vi "json To Minimized String - string path.vi"(8 "error in (no error)":errorcluster, 10 "path":string, 11 "JSON Document in":refnum<class "JSON Document.lvclass">) -> (0 "error out":errorcluster, 2 "json string":string, 3 "JSON Document out":refnum<class "JSON Document.lvclass">)   [LabVIEW 2015, in "JSON Document.lvclass"]
uses:
  JSON Document.lvclass
  JSON Document.lvclass/JSON Document.ctl
  rapidjson wrapper/rapidjson wrapper.lvlib
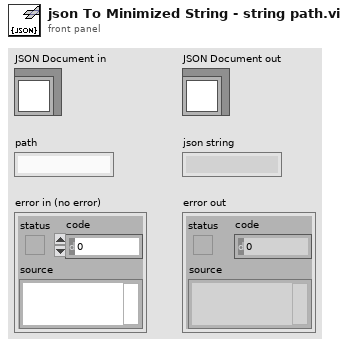
[diagram p1: front panel]
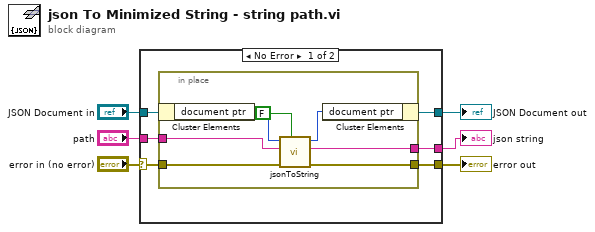
[diagram p0: block diagram]
diagram:
  n1 = case shown="No Error" "error in (no error)" {
    selector: "error in (no error)" -> [w9 w21]
    tunnel: [w8 w21] -> w5
    tunnel: [w11 w20] -> w3
    tunnel: "JSON Document in" -> [w12 w20]
    tunnel: [w10 _] -> w2
    tunnel: "path" -> [w7 _]
    frame No Error {
      n2 = in-place {
        in-place-border: [w17] -> w10
        in-place-border: w9 -> [w16]
        in-place-border: [w15] -> w8
        in-place-border: w7 -> [w14]
        n3 = in-place-cluster #1(w12) -> ("document ptr"=w19:i64)
        n4 = call "jsonToString.vi"("pretty print?"=FALSE, "error in (no error)"=w16, "path"=w14, "d in"=w19) -> ("error out"=w15:errorcluster, "json string"=w17:string, "d out"=w18:i64)  [unwired: 5 in]
        n5 = in-place-cluster #1("document ptr"=w18) -> (w11:refnum<class "JSON Document.lvclass">)
      }
    }
    frame Error {
    }
  }
  "error out" <- w5
  "JSON Document out" <- w3
  "json string" <- w2
